vi "Read Card #.vi"(8 "error in (no error)":errorcluster, 11 "Display Panel V3 in":refnum<class "Display Panel V3.lvclass">) -> (0 "error out":errorcluster, 2 "Card #":dbl, 3 "Display Panel V3 out":refnum<class "Display Panel V3.lvclass">)   [LabVIEW 2013, in "Display Panel.lvlib" / "Display Panel V3.lvclass"]
uses:
  Display Panel V3.lvclass
  Display Panel V3.lvclass/Display Panel V3.ctl
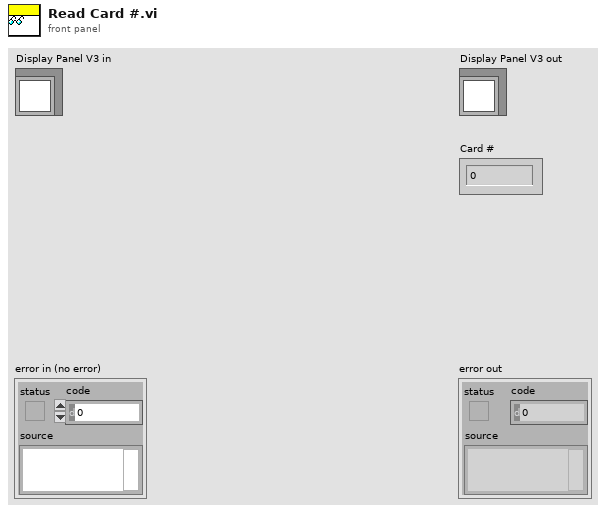
[diagram p1: front panel]
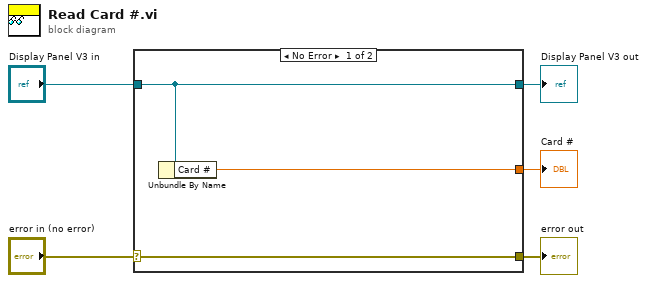
[diagram p0: block diagram]
diagram:
  n1 = case shown="No Error" "error in (no error)" {
    selector: "error in (no error)" -> [w8 w9]
    tunnel: [w8 w9] -> w4
    tunnel: [w7 w10] -> w2
    tunnel: "Display Panel V3 in" -> [w7 w10]
    tunnel: [w6 _] -> w1
    frame No Error {
      n2 = Unbundle By Name(w7) -> ("Card #"=w6:dbl)
    }
    frame Error {
    }
  }
  "error out" <- w4
  "Display Panel V3 out" <- w2
  "Card #" <- w1
